vi "BOOL2STRING.vi"(11 "Array":bool[](array[boolean])) -> (3 "String":string)   [LabVIEW 2011]
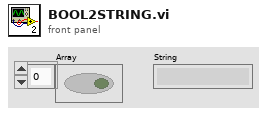
[diagram p1: front panel]
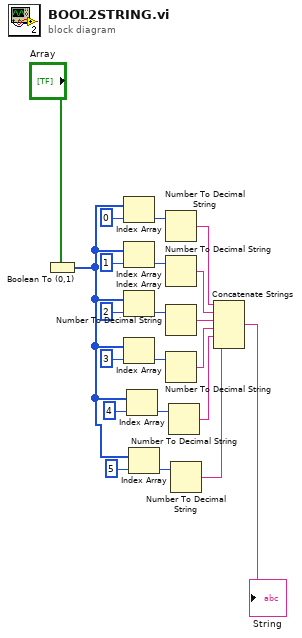
[diagram p0: block diagram]
diagram:
  n1 = Boolean To (0,1)(Boolean="Array") -> (0, 1=w19:i16[])
  n2 = Index Array(array=w19, index=0) -> (element=w5:i16)
  n3 = Index Array(array=w19, index=1) -> (element=w7:i16)
  n4 = Index Array(array=w19, index=2) -> (element=w8:i16)
  n5 = Index Array(array=w19, index=3) -> (element=w9:i16)
  n6 = Index Array(array=w19, index=4) -> (element=w16:i16)
  n7 = Index Array(array=w19, index=5) -> (element=w18:i16)
  n8 = Number To Decimal String(number=w5) -> (decimal integer string=w6:string)  [unwired: 1 in]
  n9 = Number To Decimal String(number=w7) -> (decimal integer string=w10:string)  [unwired: 1 in]
  n10 = Number To Decimal String(number=w8) -> (decimal integer string=w11:string)  [unwired: 1 in]
  n11 = Number To Decimal String(number=w9) -> (decimal integer string=w12:string)  [unwired: 1 in]
  n12 = Number To Decimal String(number=w16) -> (decimal integer string=w20:string)  [unwired: 1 in]
  n13 = Number To Decimal String(number=w18) -> (decimal integer string=w21:string)  [unwired: 1 in]
  n14 = Concatenate Strings(w6, w10, w11, w12, w20, w21) -> (→"String":string)
